vi "main.vi"(4 "function":u8(ring) items=["up", "down", "left", "right"], 5 "hum_pos in":cluster{"pos.x":i32, "pos.y":i32}, 6 "picture in":picture, 7 "image array":T1[](array[typedef]), 8 "status array in":u8[][](array[numeric])) -> (0 "hum_pos out":cluster{"pos.x":i32, "pos.y":i32}, 1 "picture out":picture, 2 "stage pass?":bool, 3 "status array out":u8[][](array[numeric]))   [LabVIEW 2018]
uses:
  <vilib>/picture/picture.llb/imagedata.ctl
  examples/LABVIEW Boxman/boxman1.03.llb/global.vi
panel:
  out "forward1":cluster{"pos.x":i32, "pos.y":i32}
  out "forward2":cluster{"pos.x":i32, "pos.y":i32}
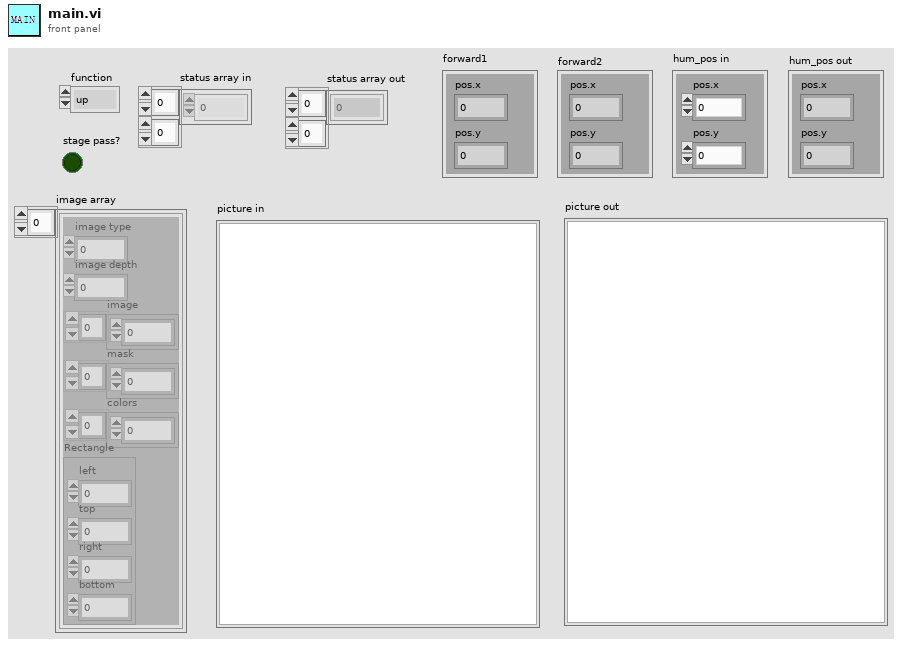
[diagram p1: front panel]
types:
  T1 = typedef "imagedata.ctl" = cluster{"image type":i32, "image depth":i32, "image":u8[], "mask":u8[], "colors":u32[], "Rectangle":cluster{"left":i16, "top":i16, "right":i16, "bottom":i16}}
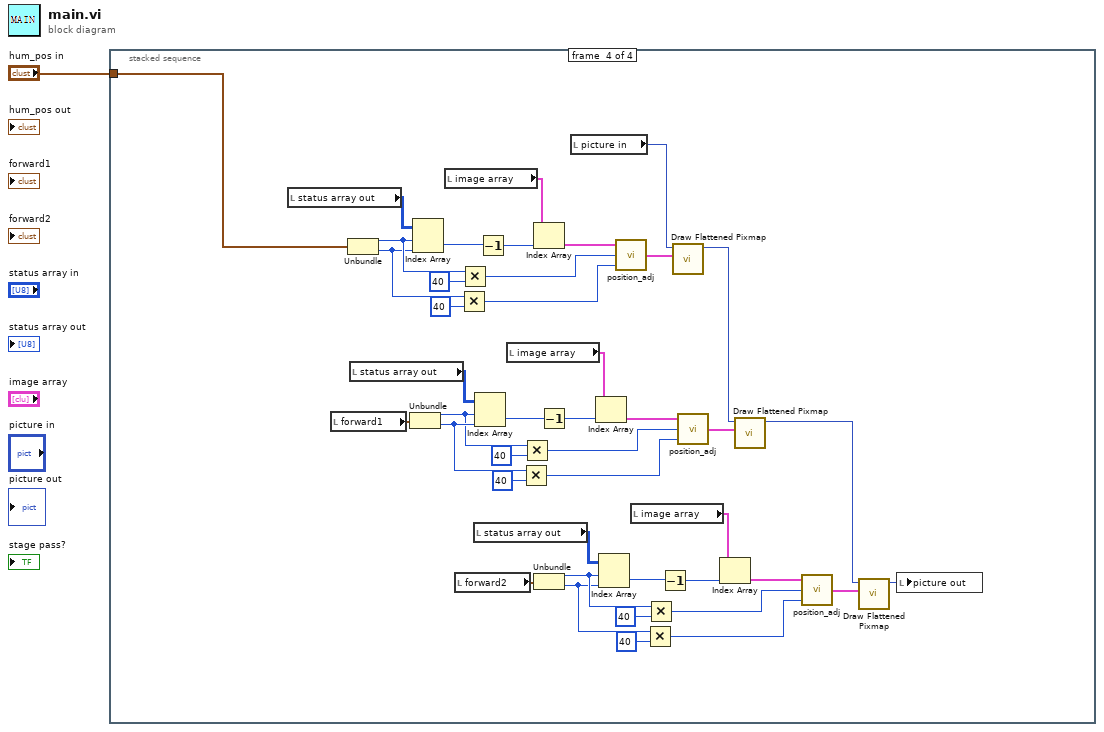
[diagram p0: block diagram]
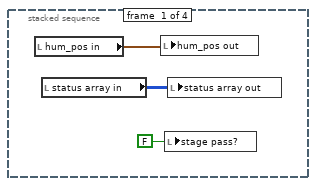
[diagram p2: hidden frame]
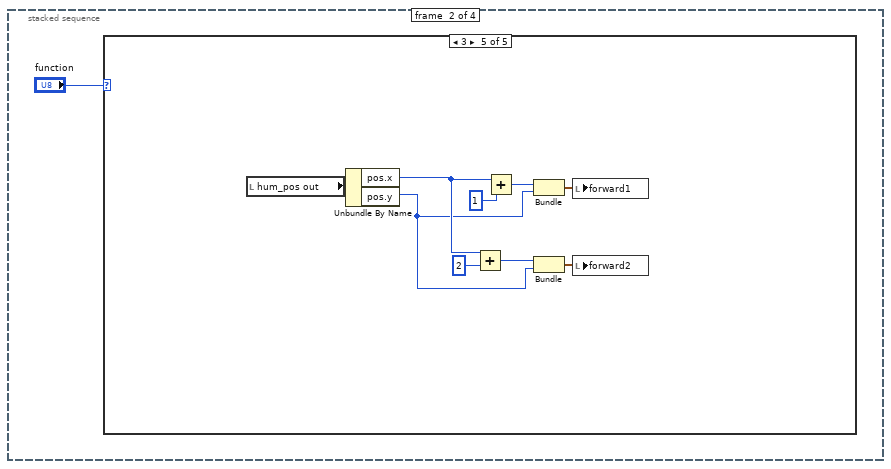
[diagram p3: hidden frame]
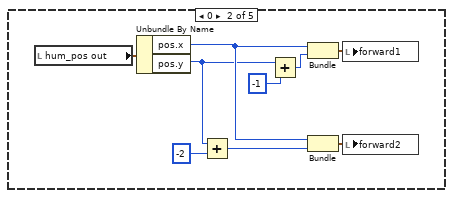
[diagram p5: hidden frame]
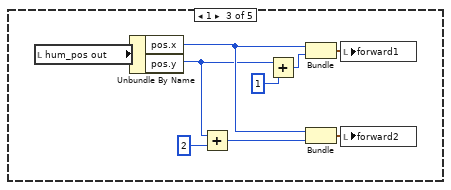
[diagram p6: hidden frame]
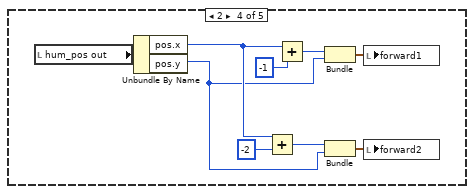
[diagram p7: hidden frame]
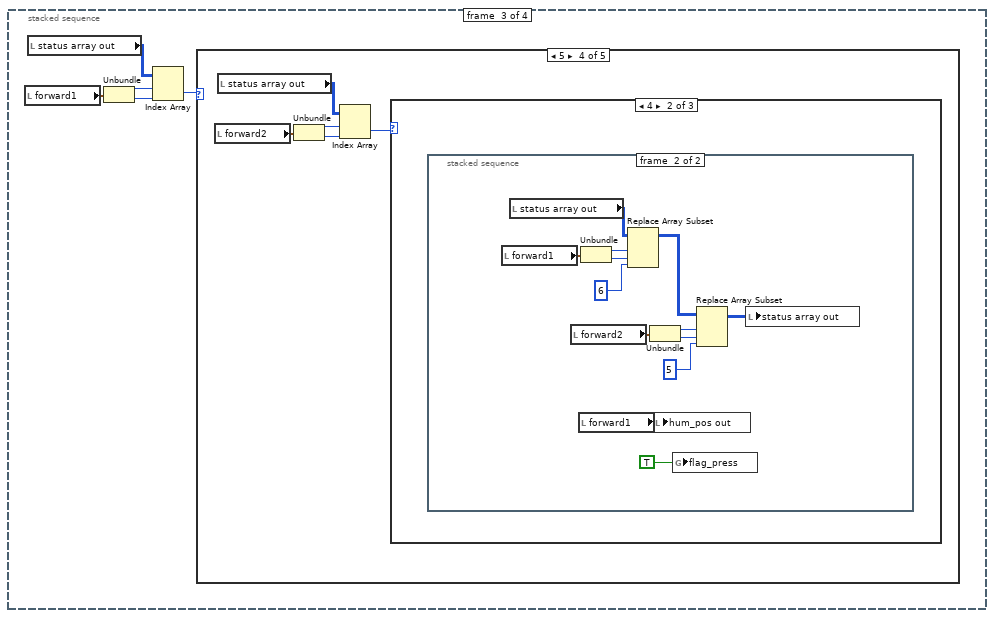
[diagram p8: hidden frame]
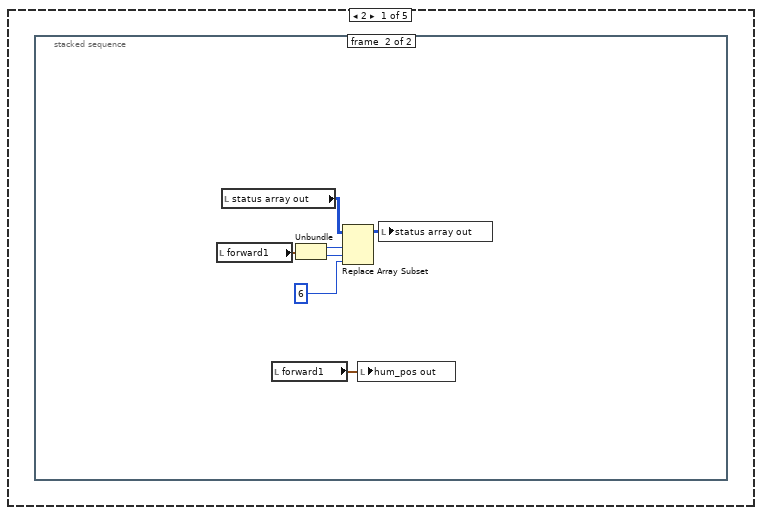
[diagram p9: hidden frame]
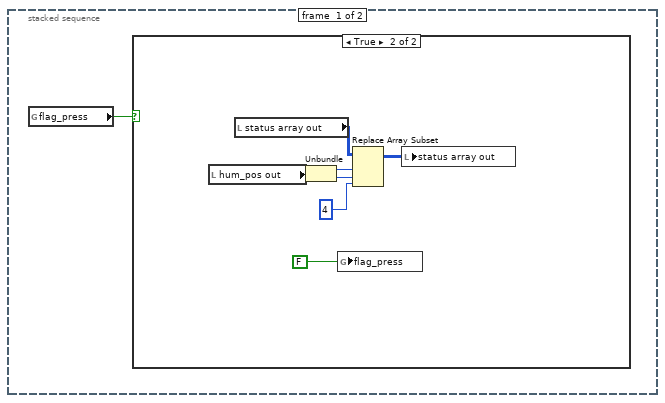
[diagram p10: hidden frame]
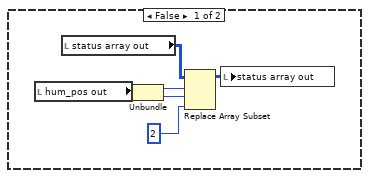
[diagram p11: hidden frame]
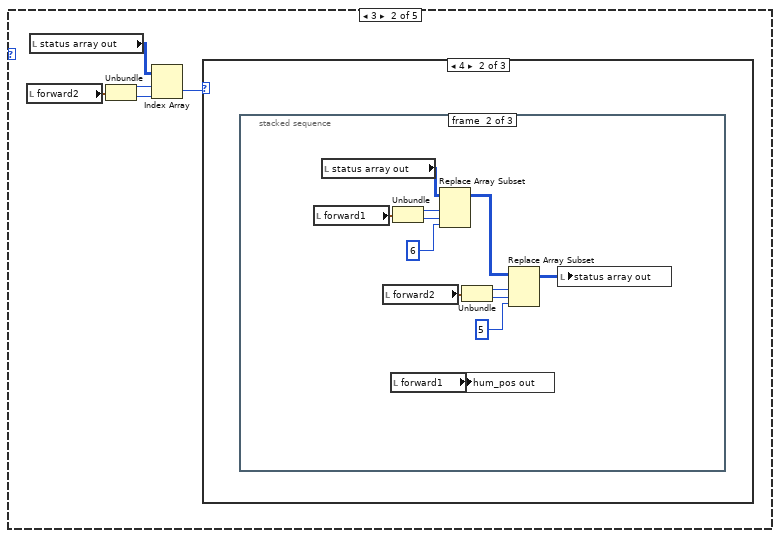
[diagram p12: hidden frame]
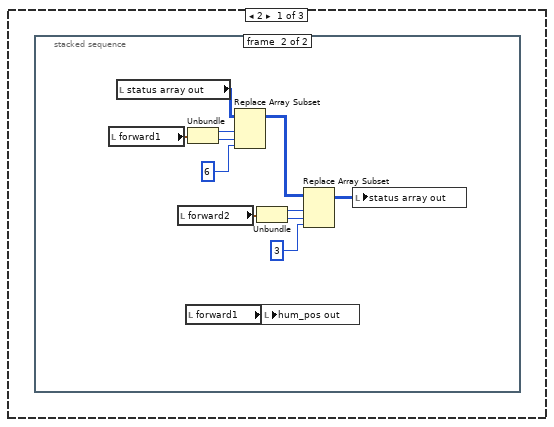
[diagram p13: hidden frame]
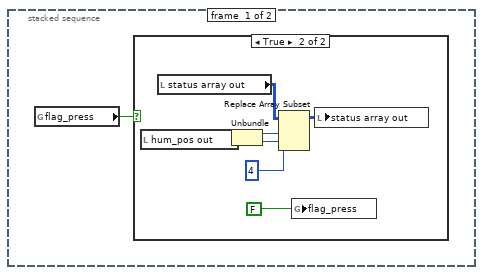
[diagram p14: hidden frame]
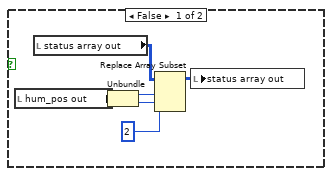
[diagram p15: hidden frame]
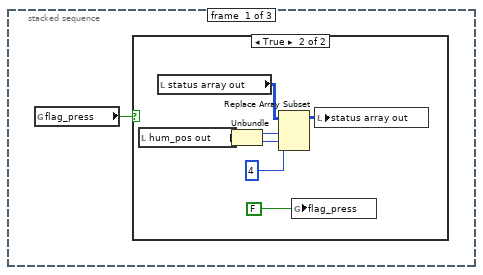
[diagram p16: hidden frame]
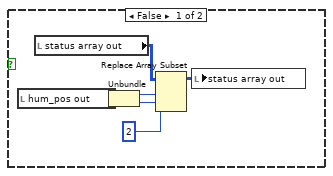
[diagram p17: hidden frame]
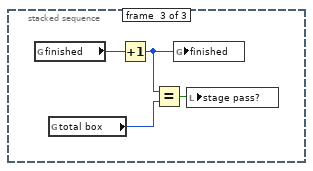
[diagram p18: hidden frame]
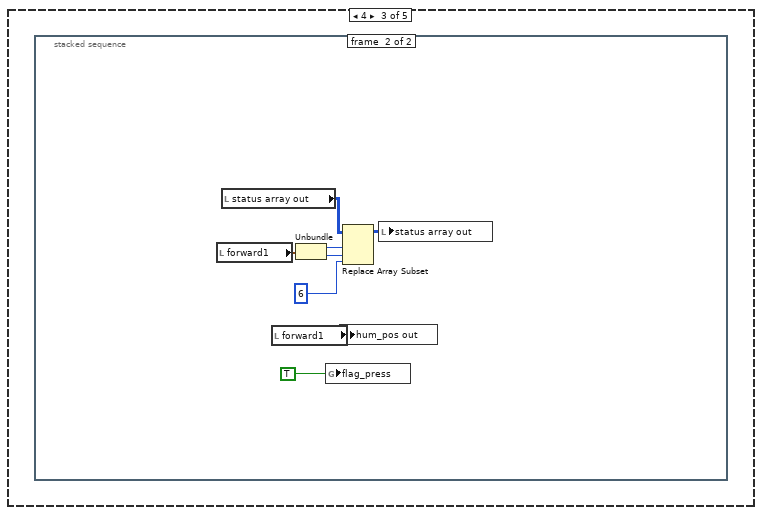
[diagram p20: hidden frame]
diagram:
  n1 = stacked-sequence {
    tunnel: "hum_pos in" -> [_ _ _ w211]
    frame #0 {
      n2 = local read "hum_pos in"() -> (w2:cluster{"pos.x":i32, "pos.y":i32})
      n3 = local read "status array in"() -> (w4:u8[][])
      n4 = local write "hum_pos out"(w2) -> ()
      n5 = local write "stage pass?"(FALSE ("stage pass?")) -> ()
      n6 = local write "status array out"(w4) -> ()
    }
    frame #1 {
      n7 = case shown="3" "function" {
        frame Default {
        }
        frame 0 {
          n8 = local read "hum_pos out"() -> (w6:cluster{"pos.x":i32, "pos.y":i32})
          n9 = Unbundle By Name(w6) -> ("pos.x"=w10:i32, "pos.y"=w7:i32)
          n10 = Add(x=w7, y=-2) -> (x+y=w12:i32)
          n11 = Add(x=w7, y=-1) -> (x+y=w9:i32)
          n12 = Bundle("pos.x"=w10, w9) -> (w14:cluster{"pos.x":i32, i32})  [unwired: 1 in]
          n13 = Bundle("pos.x"=w10, w12) -> (w11:cluster{"pos.x":i32, i32})  [unwired: 1 in]
          n14 = local write "forward1"(w14) -> ()
          n15 = local write "forward2"(w11) -> ()
        }
        frame 1 {
          n16 = local read "hum_pos out"() -> (w15:cluster{"pos.x":i32, "pos.y":i32})
          n17 = Unbundle By Name(w15) -> ("pos.x"=w19:i32, "pos.y"=w16:i32)
          n18 = Add(x=w16, y=2) -> (x+y=w21:i32)
          n19 = Add(x=w16, y=1) -> (x+y=w18:i32)
          n20 = Bundle("pos.x"=w19, w18) -> (w23:cluster{"pos.x":i32, i32})  [unwired: 1 in]
          n21 = Bundle("pos.x"=w19, w21) -> (w20:cluster{"pos.x":i32, i32})  [unwired: 1 in]
          n22 = local write "forward1"(w23) -> ()
          n23 = local write "forward2"(w20) -> ()
        }
        frame 2 {
          n24 = local read "hum_pos out"() -> (w24:cluster{"pos.x":i32, "pos.y":i32})
          n25 = Unbundle By Name(w24) -> ("pos.x"=w27:i32, "pos.y"=w25:i32)
          n26 = Add(x=w27, y=-2) -> (x+y=w26:i32)
          n27 = Add(x=w27, y=-1) -> (x+y=w28:i32)
          n28 = Bundle(w28, "pos.y"=w25) -> (w32:cluster{i32, "pos.y":i32})  [unwired: 1 in]
          n29 = Bundle(w26, "pos.y"=w25) -> (w30:cluster{i32, "pos.y":i32})  [unwired: 1 in]
          n30 = local write "forward1"(w32) -> ()
          n31 = local write "forward2"(w30) -> ()
        }
        frame 3 {
          n32 = local read "hum_pos out"() -> (w33:cluster{"pos.x":i32, "pos.y":i32})
          n33 = Unbundle By Name(w33) -> ("pos.x"=w36:i32, "pos.y"=w34:i32)
          n34 = Add(x=w36, y=2) -> (x+y=w35:i32)
          n35 = Add(x=w36, y=1) -> (x+y=w37:i32)
          n36 = Bundle(w37, "pos.y"=w34) -> (w41:cluster{i32, "pos.y":i32})  [unwired: 1 in]
          n37 = Bundle(w35, "pos.y"=w34) -> (w39:cluster{i32, "pos.y":i32})  [unwired: 1 in]
          n38 = local write "forward1"(w41) -> ()
          n39 = local write "forward2"(w39) -> ()
        }
      }
    }
    frame #2 {
      n40 = local read "forward1"() -> (w46:cluster{"pos.x":i32, "pos.y":i32})
      n41 = local read "status array out"() -> (w45:u8[][])
      n42 = Unbundle(w46) -> ("pos.x"=w44:i32, "pos.y"=w43:i32)
      n43 = Index Array(array=w45, index (row)=w44, index (col)=w43) -> (element=w42:u8)
      n44 = case shown="5" w42 {
        frame 2 {
          n45 = stacked-sequence {
            frame #0 {
              n46 = global read "global.vi" "flag_press"() -> (w47:bool)
              n47 = case shown="True" w47 {
                frame False {
                  n48 = local read "hum_pos out"() -> (w48:cluster{"pos.x":i32, "pos.y":i32})
                  n49 = local read "status array out"() -> (w53:u8[][])
                  n50 = Unbundle(w48) -> ("pos.x"=w52:i32, "pos.y"=w51:i32)
                  n51 = Replace Array Subset(array=w53, new element=u8 2 ("new element/subarray"), index (row)=w52, index (col)=w51) -> (w50:u8[][])
                  n52 = local write "status array out"(w50) -> ()
                }
                frame True {
                  n53 = local read "hum_pos out"() -> (w54:cluster{"pos.x":i32, "pos.y":i32})
                  n54 = local read "status array out"() -> (w60:u8[][])
                  n55 = Unbundle(w54) -> ("pos.x"=w59:i32, "pos.y"=w58:i32)
                  n56 = global write "global.vi" "flag_press"(FALSE) -> ()
                  n57 = Replace Array Subset(array=w60, new element=u8 4 ("new element/subarray"), index (row)=w59, index (col)=w58) -> (w57:u8[][])
                  n58 = local write "status array out"(w57) -> ()
                }
              }
            }
            frame #1 {
              n59 = local read "forward1"() -> (w66:cluster{"pos.x":i32, "pos.y":i32})
              n60 = local read "status array out"() -> (w67:u8[][])
              n61 = local read "forward1"() -> (w61:cluster{"pos.x":i32, "pos.y":i32})
              n62 = Unbundle(w66) -> ("pos.x"=w65:i32, "pos.y"=w64:i32)
              n63 = Replace Array Subset(array=w67, new element=u8 6 ("new element/subarray"), index (row)=w65, index (col)=w64) -> (w63:u8[][])
              n64 = local write "hum_pos out"(w61) -> ()
              n65 = local write "status array out"(w63) -> ()
            }
          }
        }
        frame 3 {
          n66 = local read "forward2"() -> (w69:cluster{"pos.x":i32, "pos.y":i32})
          n67 = local read "status array out"() -> (w70:u8[][])
          n68 = Unbundle(w69) -> ("pos.x"=w71:i32, "pos.y"=w72:i32)
          n69 = Index Array(array=w70, index (row)=w71, index (col)=w72) -> (element=w68:u8)
          n70 = case shown="4" w68 {
            frame 2 {
              n71 = stacked-sequence {
                frame #0 {
                  n72 = global read "global.vi" "flag_press"() -> (w73:bool)
                  n73 = case shown="True" w73 {
                    frame False {
                      n74 = local read "hum_pos out"() -> (w74:cluster{"pos.x":i32, "pos.y":i32})
                      n75 = local read "status array out"() -> (w79:u8[][])
                      n76 = Unbundle(w74) -> ("pos.x"=w78:i32, "pos.y"=w77:i32)
                      n77 = Replace Array Subset(array=w79, new element=u8 2 ("new element/subarray"), index (row)=w78, index (col)=w77) -> (w76:u8[][])
                      n78 = local write "status array out"(w76) -> ()
                    }
                    frame True {
                      n79 = local read "hum_pos out"() -> (w80:cluster{"pos.x":i32, "pos.y":i32})
                      n80 = local read "status array out"() -> (w86:u8[][])
                      n81 = Unbundle(w80) -> ("pos.x"=w85:i32, "pos.y"=w84:i32)
                      n82 = Replace Array Subset(array=w86, new element=u8 4 ("new element/subarray"), index (row)=w85, index (col)=w84) -> (w83:u8[][])
                      n83 = global write "global.vi" "flag_press"(FALSE) -> ()
                      n84 = local write "status array out"(w83) -> ()
                    }
                  }
                }
                frame #1 {
                  n85 = local read "forward1"() -> (w97:cluster{"pos.x":i32, "pos.y":i32})
                  n86 = local read "status array out"() -> (w98:u8[][])
                  n87 = local read "forward2"() -> (w90:cluster{"pos.x":i32, "pos.y":i32})
                  n88 = local read "forward1"() -> (w87:cluster{"pos.x":i32, "pos.y":i32})
                  n89 = Unbundle(w97) -> ("pos.x"=w96:i32, "pos.y"=w95:i32)
                  n90 = Replace Array Subset(array=w98, new element=u8 6 ("new element/subarray"), index (row)=w96, index (col)=w95) -> (w88:u8[][])
                  n91 = Unbundle(w90) -> ("pos.x"=w91:i32, "pos.y"=w92:i32)
                  n92 = local write "hum_pos out"(w87) -> ()
                  n93 = Replace Array Subset(array=w88, new element=u8 3 ("new element/subarray"), index (row)=w91, index (col)=w92) -> (w93:u8[][])
                  n94 = local write "status array out"(w93) -> ()
                }
              }
            }
            frame 4 {
              n95 = stacked-sequence {
                frame #0 {
                  n96 = global read "global.vi" "flag_press"() -> (w99:bool)
                  n97 = case shown="True" w99 {
                    frame False {
                      n98 = local read "hum_pos out"() -> (w100:cluster{"pos.x":i32, "pos.y":i32})
                      n99 = local read "status array out"() -> (w105:u8[][])
                      n100 = Unbundle(w100) -> ("pos.x"=w104:i32, "pos.y"=w103:i32)
                      n101 = Replace Array Subset(array=w105, new element=u8 2 ("new element/subarray"), index (row)=w104, index (col)=w103) -> (w102:u8[][])
                      n102 = local write "status array out"(w102) -> ()
                    }
                    frame True {
                      n103 = local read "hum_pos out"() -> (w106:cluster{"pos.x":i32, "pos.y":i32})
                      n104 = local read "status array out"() -> (w112:u8[][])
                      n105 = Unbundle(w106) -> ("pos.x"=w111:i32, "pos.y"=w110:i32)
                      n106 = Replace Array Subset(array=w112, new element=u8 4 ("new element/subarray"), index (row)=w111, index (col)=w110) -> (w109:u8[][])
                      n107 = global write "global.vi" "flag_press"(FALSE) -> ()
                      n108 = local write "status array out"(w109) -> ()
                    }
                  }
                }
                frame #1 {
                  n109 = local read "forward1"() -> (w123:cluster{"pos.x":i32, "pos.y":i32})
                  n110 = local read "status array out"() -> (w124:u8[][])
                  n111 = local read "forward2"() -> (w116:cluster{"pos.x":i32, "pos.y":i32})
                  n112 = local read "forward1"() -> (w113:cluster{"pos.x":i32, "pos.y":i32})
                  n113 = Unbundle(w123) -> ("pos.x"=w122:i32, "pos.y"=w121:i32)
                  n114 = Replace Array Subset(array=w124, new element=u8 6 ("new element/subarray"), index (row)=w122, index (col)=w121) -> (w114:u8[][])
                  n115 = local write "hum_pos out"(w113) -> ()
                  n116 = Unbundle(w116) -> ("pos.x"=w117:i32, "pos.y"=w118:i32)
                  n117 = Replace Array Subset(array=w114, new element=u8 5 ("new element/subarray"), index (row)=w117, index (col)=w118) -> (w119:u8[][])
                  n118 = local write "status array out"(w119) -> ()
                }
                frame #2 {
                  n119 = global read "global.vi" "finished"() -> (w128:u32)
                  n120 = global read "global.vi" "total box"() -> (w126:u32)
                  n121 = Increment(x=w128) -> (x+1=w127:u32)
                  n122 = Equal?(x=w127, y=w126) -> (x = y?=w125:bool)
                  n123 = global write "global.vi" "finished"(w127) -> ()
                  n124 = local write "stage pass?"(w125) -> ()
                }
              }
            }
            frame Default {
            }
          }
        }
        frame 4 {
          n125 = stacked-sequence {
            frame #0 {
              n126 = global read "global.vi" "flag_press"() -> (w129:bool)
              n127 = case shown="True" w129 {
                frame False {
                  n128 = local read "hum_pos out"() -> (w130:cluster{"pos.x":i32, "pos.y":i32})
                  n129 = local read "status array out"() -> (w135:u8[][])
                  n130 = Unbundle(w130) -> ("pos.x"=w134:i32, "pos.y"=w133:i32)
                  n131 = Replace Array Subset(array=w135, new element=u8 2 ("new element/subarray"), index (row)=w134, index (col)=w133) -> (w132:u8[][])
                  n132 = local write "status array out"(w132) -> ()
                }
                frame True {
                  n133 = local read "hum_pos out"() -> (w136:cluster{"pos.x":i32, "pos.y":i32})
                  n134 = local read "status array out"() -> (w141:u8[][])
                  n135 = Unbundle(w136) -> ("pos.x"=w140:i32, "pos.y"=w139:i32)
                  n136 = Replace Array Subset(array=w141, new element=u8 4 ("new element/subarray"), index (row)=w140, index (col)=w139) -> (w138:u8[][])
                  n137 = local write "status array out"(w138) -> ()
                }
              }
            }
            frame #1 {
              n138 = local read "forward1"() -> (w148:cluster{"pos.x":i32, "pos.y":i32})
              n139 = local read "status array out"() -> (w149:u8[][])
              n140 = local read "forward1"() -> (w142:cluster{"pos.x":i32, "pos.y":i32})
              n141 = Unbundle(w148) -> ("pos.x"=w147:i32, "pos.y"=w146:i32)
              n142 = global write "global.vi" "flag_press"(TRUE) -> ()
              n143 = local write "hum_pos out"(w142) -> ()
              n144 = Replace Array Subset(array=w149, new element=u8 6 ("new element/subarray"), index (row)=w147, index (col)=w146) -> (w145:u8[][])
              n145 = local write "status array out"(w145) -> ()
            }
          }
        }
        frame 5 {
          n146 = local read "forward2"() -> (w151:cluster{"pos.x":i32, "pos.y":i32})
          n147 = local read "status array out"() -> (w152:u8[][])
          n148 = Unbundle(w151) -> ("pos.x"=w153:i32, "pos.y"=w154:i32)
          n149 = Index Array(array=w152, index (row)=w153, index (col)=w154) -> (element=w150:u8)
          n150 = case shown="4" w150 {
            frame 2 {
              n151 = stacked-sequence {
                frame #0 {
                  n152 = global read "global.vi" "flag_press"() -> (w155:bool)
                  n153 = case shown="True" w155 {
                    frame False {
                      n154 = local read "hum_pos out"() -> (w156:cluster{"pos.x":i32, "pos.y":i32})
                      n155 = local read "status array out"() -> (w161:u8[][])
                      n156 = Unbundle(w156) -> ("pos.x"=w160:i32, "pos.y"=w159:i32)
                      n157 = Replace Array Subset(array=w161, new element=u8 2 ("new element/subarray"), index (row)=w160, index (col)=w159) -> (w158:u8[][])
                      n158 = local write "status array out"(w158) -> ()
                    }
                    frame True {
                      n159 = local read "hum_pos out"() -> (w162:cluster{"pos.x":i32, "pos.y":i32})
                      n160 = local read "status array out"() -> (w168:u8[][])
                      n161 = Unbundle(w162) -> ("pos.x"=w167:i32, "pos.y"=w166:i32)
                      n162 = Replace Array Subset(array=w168, new element=u8 4 ("new element/subarray"), index (row)=w167, index (col)=w166) -> (w165:u8[][])
                      n163 = global write "global.vi" "flag_press"(FALSE) -> ()
                      n164 = local write "status array out"(w165) -> ()
                    }
                  }
                }
                frame #1 {
                  n165 = local read "forward1"() -> (w182:cluster{"pos.x":i32, "pos.y":i32})
                  n166 = local read "status array out"() -> (w183:u8[][])
                  n167 = local read "forward2"() -> (w175:cluster{"pos.x":i32, "pos.y":i32})
                  n168 = local read "forward1"() -> (w169:cluster{"pos.x":i32, "pos.y":i32})
                  n169 = Unbundle(w182) -> ("pos.x"=w181:i32, "pos.y"=w180:i32)
                  n170 = global read "global.vi" "finished"() -> (w171:u32)
                  n171 = global write "global.vi" "flag_press"(TRUE ("flag_press")) -> ()
                  n172 = Replace Array Subset(array=w183, new element=u8 6 ("new element/subarray"), index (row)=w181, index (col)=w180) -> (w173:u8[][])
                  n173 = local write "hum_pos out"(w169) -> ()
                  n174 = Unbundle(w175) -> ("pos.x"=w176:i32, "pos.y"=w177:i32)
                  n175 = Decrement(x=w171) -> (x-1=w170:u32)
                  n176 = Replace Array Subset(array=w173, new element=u8 3 ("new element/subarray"), index (row)=w176, index (col)=w177) -> (w178:u8[][])
                  n177 = global write "global.vi" "finished"(w170) -> ()
                  n178 = local write "status array out"(w178) -> ()
                }
              }
            }
            frame 4 {
              n179 = stacked-sequence {
                frame #0 {
                  n180 = global read "global.vi" "flag_press"() -> (w184:bool)
                  n181 = case shown="True" w184 {
                    frame False {
                      n182 = local read "hum_pos out"() -> (w185:cluster{"pos.x":i32, "pos.y":i32})
                      n183 = local read "status array out"() -> (w190:u8[][])
                      n184 = Unbundle(w185) -> ("pos.x"=w189:i32, "pos.y"=w188:i32)
                      n185 = Replace Array Subset(array=w190, new element=u8 2 ("new element/subarray"), index (row)=w189, index (col)=w188) -> (w187:u8[][])
                      n186 = local write "status array out"(w187) -> ()
                    }
                    frame True {
                      n187 = local read "hum_pos out"() -> (w191:cluster{"pos.x":i32, "pos.y":i32})
                      n188 = local read "status array out"() -> (w197:u8[][])
                      n189 = Unbundle(w191) -> ("pos.x"=w196:i32, "pos.y"=w195:i32)
                      n190 = Replace Array Subset(array=w197, new element=u8 4 ("new element/subarray"), index (row)=w196, index (col)=w195) -> (w194:u8[][])
                      n191 = global write "global.vi" "flag_press"(FALSE) -> ()
                      n192 = local write "status array out"(w194) -> ()
                    }
                  }
                }
                frame #1 {
                  n193 = local read "forward1"() -> (w209:cluster{"pos.x":i32, "pos.y":i32})
                  n194 = local read "status array out"() -> (w210:u8[][])
                  n195 = local read "forward2"() -> (w202:cluster{"pos.x":i32, "pos.y":i32})
                  n196 = local read "forward1"() -> (w198:cluster{"pos.x":i32, "pos.y":i32})
                  n197 = Unbundle(w209) -> ("pos.x"=w208:i32, "pos.y"=w207:i32)
                  n198 = Replace Array Subset(array=w210, new element=u8 6 ("new element/subarray"), index (row)=w208, index (col)=w207) -> (w200:u8[][])
                  n199 = Unbundle(w202) -> ("pos.x"=w203:i32, "pos.y"=w204:i32)
                  n200 = local write "hum_pos out"(w198) -> ()
                  n201 = global write "global.vi" "flag_press"(TRUE ("flag_press")) -> ()
                  n202 = Replace Array Subset(array=w200, new element=u8 5 ("new element/subarray"), index (row)=w203, index (col)=w204) -> (w205:u8[][])
                  n203 = local write "status array out"(w205) -> ()
                }
              }
            }
            frame Default {
            }
          }
        }
        frame Default {
        }
      }
    }
    frame #3 {
      n204 = local read "status array out"() -> (w250:u8[][])
      n205 = local read "forward1"() -> (w234:cluster{"pos.x":i32, "pos.y":i32})
      n206 = Unbundle(w211) -> ("pos.x"=w247:i32, "pos.y"=w246:i32)
      n207 = local read "status array out"() -> (w235:u8[][])
      n208 = Unbundle(w234) -> ("pos.x"=w238:i32, "pos.y"=w239:i32)
      n209 = Index Array(array=w250, index (row)=w247, index (col)=w246) -> (element=w217:u8)
      n210 = local read "image array"() -> (w249:T1[])
      n211 = local read "forward2"() -> (w229:cluster{"pos.x":i32, "pos.y":i32})
      n212 = Multiply(x=w246, y=40) -> (x*y=w244:i32)
      n213 = Multiply(x=w247, y=40) -> (x*y=w245:i32)
      n214 = local read "status array out"() -> (w228:u8[][])
      n215 = Index Array(array=w235, index (row)=w238, index (col)=w239) -> (element=w215:u8)
      n216 = Decrement(x=w217) -> (x-1=w216:u8)
      n217 = local read "image array"() -> (w236:T1[])
      n218 = Multiply(x=w239, y=40) -> (x*y=w241:i32)
      n219 = Multiply(x=w238, y=40) -> (x*y=w240:i32)
      n220 = Index Array(array=w249, index=w216) -> (element=w248:T1)
      n221 = Unbundle(w229) -> ("pos.x"=w225:i32, "pos.y"=w224:i32)
      n222 = Decrement(x=w215) -> (x-1=w214:u8)
      n223 = local read "picture in"() -> (w253:picture)
      n224 = Index Array(array=w236, index=w214) -> (element=w237:T1)
      n225 = Index Array(array=w228, index (row)=w225, index (col)=w224) -> (element=w213:u8)
      n226 = call "position_adj.vi"("coordinate.y"=w244, "coordinate.x"=w245, "image data in"=w248) -> ("image data out"=w243:T1)
      n227 = local read "image array"() -> (w227:T1[])
      n228 = Multiply(x=w224, y=40) -> (x*y=w222:i32)
      n229 = Multiply(x=w225, y=40) -> (x*y=w223:i32)
      n230 = Decrement(x=w213) -> (x-1=w212:u8)
      n231 = call <vilib>:"Draw Flattened Pixmap.vi"("image data"=w243, "picture"=w253) -> ("new picture"=w220:picture)  [unwired: 7 in]
      n232 = call "position_adj.vi"("coordinate.y"=w241, "coordinate.x"=w240, "image data in"=w237) -> ("image data out"=w242:T1)
      n233 = Index Array(array=w227, index=w212) -> (element=w226:T1)
      n234 = call <vilib>:"Draw Flattened Pixmap.vi"("image data"=w242, "picture"=w220) -> ("new picture"=w219:picture)  [unwired: 7 in]
      n235 = call "position_adj.vi"("coordinate.y"=w222, "coordinate.x"=w223, "image data in"=w226) -> ("image data out"=w221:T1)
      n236 = call <vilib>:"Draw Flattened Pixmap.vi"("image data"=w221, "picture"=w219) -> ("new picture"=w218:picture)  [unwired: 7 in]
      n237 = local write "picture out"(w218) -> ()
    }
  }
